vi "Remove all hyphens in string.vi"(4 "MAC Address":string="AA-BB-CC-DD-EE-FF") -> (1 "result string":string)   [LabVIEW 2020]
uses:
  <vilib>/Utility/error.llb/whitespace.ctl
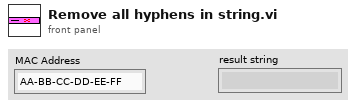
[diagram p1: front panel]
types:
  T1 = typedef "whitespace.ctl" = u16
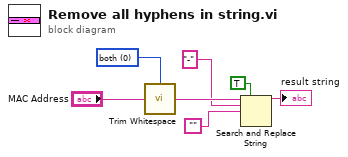
[diagram p0: block diagram]
diagram:
  w7 = T1 0 items=["both", "start of string", "end of string"] ("location (both)")
  n1 = call <vilib>:"Trim Whitespace.vi"("string"="MAC Address", "location (both)"=w7) -> ("trimmed string"=w6:string)
  n2 = Search and Replace String(replace all?=TRUE ("replace all? (F)"), input string=w6, search string="-", replace string="") -> (result string=→"result string":string)  [unwired: 4 in, 3 out]
